vi "Lab Panel V5.22.vi"() -> ()   [LabVIEW 2013] (continued)
                      frame #0 {
                        n2184 = case shown="True" w3895 {
                          tunnel: w3894 -> [_ w3900]
                          tunnel: w3893 -> [_ w3899]
                          tunnel: w3892 -> [_ w3898]
                          tunnel: w3891 -> [_ w3896]
                          frame False {
                          }
                          frame True {
                            n2185 = Bundle(cluster=w3896, "amps"=w3900, "volts"=w3899, "pf"=w3898) -> (w3897:cluster{"amps":dbl, "volts":dbl, "pf":dbl})
                            n2186 = local write "ON L01-1"(w3897) -> ()
                          }
                        }
                      }
                      frame #1 {
                        n2187 = Unbundle(w3905) -> ("amps"=w3904:dbl, "volts"=w3903:dbl, "pf"=w3902:dbl)
                        n2188 = case shown="True" w3906 {
                          tunnel: w3913 -> [_ w3914]
                          tunnel: w3912 -> [_ w3952]
                          tunnel: w3911 -> [_ _]
                          tunnel: w3910 -> [_ _]
                          tunnel: w3909 -> [_ w3951]
                          tunnel: w3908 -> [_ w3950]
                          tunnel: w3907 -> [_ w3918]
                          tunnel: w3904 -> [_ w3915]
                          tunnel: w3903 -> [_ w3947]
                          tunnel: w3902 -> [_ w3946]
                          tunnel: w3901 -> [_ w3916]
                          frame False {
                          }
                          frame True {
                            n2189 = local read "TDMS LAB01-1"() -> (w3949:refnum<k34>)
                            n2190 = Build Array(w3947) -> (w3943:dbl[])
                            n2191 = Build Array(w3946) -> (w3942:dbl[])
                            n2192 = Build Array(w3951) -> (w3941:dbl[])
                            n2193 = Build Array(w3952) -> (w3940:dbl[])
                            n2194 = Build Array(w3915) -> (w3945:dbl[])
                            n2195 = Build Array(w3914) -> (w3944:dbl[])
                            n2196 = Build Array(w3950) -> (w3939:dbl[])
                            n2197 = Build Array("AMPS ON", "AMPS OFF", "VOLTS", "PF", "TEMP Live", "TEMP Neut", "CYCLE") -> (w3923:string[])
                            n2198 = Bundle By Name("Y"=w3945, "t0"=w3916) -> (w3938:waveform(dbl))  [unwired: 1 in]
                            n2199 = Bundle By Name("Y"=w3944, "t0"=w3916) -> (w3937:waveform(dbl))  [unwired: 1 in]
                            n2200 = Bundle By Name("Y"=w3943, "t0"=w3916) -> (w3936:waveform(dbl))  [unwired: 1 in]
                            n2201 = Bundle By Name("Y"=w3942, "t0"=w3916) -> (w3935:waveform(dbl))  [unwired: 1 in]
                            n2202 = Bundle By Name("Y"=w3941, "t0"=w3916) -> (w3934:waveform(dbl))  [unwired: 1 in]
                            n2203 = Bundle By Name("Y"=w3940, "t0"=w3916) -> (w3933:waveform(dbl))  [unwired: 1 in]
                            n2204 = Bundle By Name("Y"=w3939, "t0"=w3916) -> (w3932:waveform(dbl))  [unwired: 1 in]
                            n2205 = Build Array(w3938, w3937, w3936, w3935, w3934, w3933, w3932) -> (w3931:waveform(dbl)[])
                            n2206 = TDMS Write(0:w3949, 5:"TEST VALUES", 7:w3923, 9:w3931) -> (4:w3922:refnum<k34>, 6:w3921:string, 15:w3920:errorcluster)  [unwired: 2 in, 1 out]
                            n2207 = TDMS Write(0:w3922, 5:w3921, 7:"TIME", 9:w3918, 11:w3920) -> (15:w3917:errorcluster)  [unwired: 1 in, 3 out]
                            n2208 = local write "data file error"(w3917) -> ()
                          }
                        }
                      }
                    }
                  }
                }
              }
              frame #1 {
                n2209 = case shown="True" w3953 {
                  tunnel: w3957 -> [_ w3962]
                  tunnel: w3956 -> [_ w3961]
                  tunnel: w3955 -> [_ w3959]
                  tunnel: w3954 -> [_ w3958]
                  frame False {
                  }
                  frame True {
                    n2210 = local read "DISP LAB01-2"() -> (w3963:T4)
                    n2211 = local read "SIG LAB01-2"() -> (w3964:T2)
                    n2212 = local read "ON L01-2"() -> (w3960:cluster{"amps":dbl, "volts":dbl, "pf":dbl})
                    n2213 = Unbundle(w3964) -> ("AMPS"=w3970:dbl, "VOLTS"=w3968:dbl, "PF"=w3967:dbl, "Tmp Live"=w3966:dbl, "Tmp Neut"=w3969:dbl)
                    n2214 = Unbundle(w3963) -> ("CYCLE"=w3965:dbl)  [unwired: 2 out]
                    n2215 = stacked-sequence {
                      tunnel: w3970 -> [w3974 w3993]
                      tunnel: w3969 -> [_ w3992]
                      tunnel: w3968 -> [w3973 w3991]
                      tunnel: w3967 -> [w3972 w3990]
                      tunnel: w3966 -> [_ w3989]
                      tunnel: w3965 -> [_ w3988]
                      tunnel: w3962 -> [_ w3987]
                      tunnel: w3961 -> [w3975 _]
                      tunnel: w3960 -> [w3971 w3985]
                      tunnel: w3959 -> [_ w3986]
                      tunnel: w3958 -> [_ w3981]
                      frame #0 {
                        n2216 = case shown="True" w3975 {
                          tunnel: w3974 -> [_ w3980]
                          tunnel: w3973 -> [_ w3979]
                          tunnel: w3972 -> [_ w3978]
                          tunnel: w3971 -> [_ w3976]
                          frame False {
                          }
                          frame True {
                            n2217 = Bundle(cluster=w3976, "amps"=w3980, "volts"=w3979, "pf"=w3978) -> (w3977:cluster{"amps":dbl, "volts":dbl, "pf":dbl})
                            n2218 = local write "ON L01-2"(w3977) -> ()
                          }
                        }
                      }
                      frame #1 {
                        n2219 = Unbundle(w3985) -> ("amps"=w3984:dbl, "volts"=w3983:dbl, "pf"=w3982:dbl)
                        n2220 = case shown="True" w3986 {
                          tunnel: w3993 -> [_ w4025]
                          tunnel: w3992 -> [_ w4032]
                          tunnel: w3991 -> [_ _]
                          tunnel: w3990 -> [_ _]
                          tunnel: w3989 -> [_ w4031]
                          tunnel: w3988 -> [_ w4030]
                          tunnel: w3987 -> [_ w3995]
                          tunnel: w3984 -> [_ w4027]
                          tunnel: w3983 -> [_ w4026]
                          tunnel: w3982 -> [_ w4024]
                          tunnel: w3981 -> [_ w4016]
                          frame False {
                          }
                          frame True {
                            n2221 = local read "TDMS LAB01-2"() -> (w4029:refnum<k34>)
                            n2222 = Build Array(w4026) -> (w4021:dbl[])
                            n2223 = Build Array(w4024) -> (w4020:dbl[])
                            n2224 = Build Array(w4031) -> (w4019:dbl[])
                            n2225 = Build Array(w4032) -> (w4018:dbl[])
                            n2226 = Build Array(w4027) -> (w4023:dbl[])
                            n2227 = Build Array(w4025) -> (w4022:dbl[])
                            n2228 = Build Array(w4030) -> (w4017:dbl[])
                            n2229 = Build Array("AMPS ON", "AMPS OFF", "VOLTS", "PF", "TEMP Live", "TEMP Neut", "CYCLE") -> (w4000:string[])
                            n2230 = Bundle By Name("Y"=w4023, "t0"=w4016) -> (w4015:waveform(dbl))  [unwired: 1 in]
                            n2231 = Bundle By Name("Y"=w4022, "t0"=w4016) -> (w4014:waveform(dbl))  [unwired: 1 in]
                            n2232 = Bundle By Name("Y"=w4021, "t0"=w4016) -> (w4013:waveform(dbl))  [unwired: 1 in]
                            n2233 = Bundle By Name("Y"=w4020, "t0"=w4016) -> (w4012:waveform(dbl))  [unwired: 1 in]
                            n2234 = Bundle By Name("Y"=w4019, "t0"=w4016) -> (w4011:waveform(dbl))  [unwired: 1 in]
                            n2235 = Bundle By Name("Y"=w4018, "t0"=w4016) -> (w4010:waveform(dbl))  [unwired: 1 in]
                            n2236 = Bundle By Name("Y"=w4017, "t0"=w4016) -> (w4009:waveform(dbl))  [unwired: 1 in]
                            n2237 = Build Array(w4015, w4014, w4013, w4012, w4011, w4010, w4009) -> (w4008:waveform(dbl)[])
                            n2238 = TDMS Write(0:w4029, 5:"TEST VALUES", 7:w4000, 9:w4008) -> (4:w3999:refnum<k34>, 6:w3998:string, 15:w3997:errorcluster)  [unwired: 2 in, 1 out]
                            n2239 = TDMS Write(0:w3999, 5:w3998, 7:"TIME", 9:w3995, 11:w3997) -> (15:w3994:errorcluster)  [unwired: 1 in, 3 out]
                            n2240 = local write "data file error"(w3994) -> ()
                          }
                        }
                      }
                    }
                  }
                }
              }
              frame #2 {
                n2241 = case shown="True" w4033 {
                  tunnel: w4037 -> [_ w4042]
                  tunnel: w4036 -> [_ w4041]
                  tunnel: w4035 -> [_ w4039]
                  tunnel: w4034 -> [_ w4038]
                  frame False {
                  }
                  frame True {
                    n2242 = local read "DISP LAB02-1"() -> (w4043:T4)
                    n2243 = local read "SIG LAB02-1"() -> (w4044:T2)
                    n2244 = local read "ON L02-1"() -> (w4040:cluster{"amps":dbl, "volts":dbl, "pf":dbl})
                    n2245 = Unbundle(w4044) -> ("AMPS"=w4050:dbl, "VOLTS"=w4048:dbl, "PF"=w4047:dbl, "Tmp Live"=w4046:dbl, "Tmp Neut"=w4049:dbl)
                    n2246 = Unbundle(w4043) -> ("CYCLE"=w4045:dbl)  [unwired: 2 out]
                    n2247 = stacked-sequence {
                      tunnel: w4050 -> [w4054 w4073]
                      tunnel: w4049 -> [_ w4072]
                      tunnel: w4048 -> [w4053 w4071]
                      tunnel: w4047 -> [w4052 w4070]
                      tunnel: w4046 -> [_ w4069]
                      tunnel: w4045 -> [_ w4068]
                      tunnel: w4042 -> [_ w4067]
                      tunnel: w4041 -> [w4055 _]
                      tunnel: w4040 -> [w4051 w4065]
                      tunnel: w4039 -> [_ w4066]
                      tunnel: w4038 -> [_ w4061]
                      frame #0 {
                        n2248 = case shown="True" w4055 {
                          tunnel: w4054 -> [_ w4060]
                          tunnel: w4053 -> [_ w4059]
                          tunnel: w4052 -> [_ w4058]
                          tunnel: w4051 -> [_ w4056]
                          frame False {
                          }
                          frame True {
                            n2249 = Bundle(cluster=w4056, "amps"=w4060, "volts"=w4059, "pf"=w4058) -> (w4057:cluster{"amps":dbl, "volts":dbl, "pf":dbl})
                            n2250 = local write "ON L02-1"(w4057) -> ()
                          }
                        }
                      }
                      frame #1 {
                        n2251 = Unbundle(w4065) -> ("amps"=w4064:dbl, "volts"=w4063:dbl, "pf"=w4062:dbl)
                        n2252 = case shown="True" w4066 {
                          tunnel: w4073 -> [_ w4105]
                          tunnel: w4072 -> [_ w4112]
                          tunnel: w4071 -> [_ _]
                          tunnel: w4070 -> [_ _]
                          tunnel: w4069 -> [_ w4111]
                          tunnel: w4068 -> [_ w4110]
                          tunnel: w4067 -> [_ w4075]
                          tunnel: w4064 -> [_ w4107]
                          tunnel: w4063 -> [_ w4106]
                          tunnel: w4062 -> [_ w4104]
                          tunnel: w4061 -> [_ w4096]
                          frame False {
                          }
                          frame True {
                            n2253 = local read "TDMS LAB02-1"() -> (w4109:refnum<k34>)
                            n2254 = Build Array(w4106) -> (w4101:dbl[])
                            n2255 = Build Array(w4104) -> (w4100:dbl[])
                            n2256 = Build Array(w4111) -> (w4099:dbl[])
                            n2257 = Build Array(w4112) -> (w4098:dbl[])
                            n2258 = Build Array(w4107) -> (w4103:dbl[])
                            n2259 = Build Array(w4105) -> (w4102:dbl[])
                            n2260 = Build Array(w4110) -> (w4097:dbl[])
                            n2261 = Build Array("AMPS ON", "AMPS OFF", "VOLTS", "PF", "TEMP Live", "TEMP Neut", "CYCLE") -> (w4080:string[])
                            n2262 = Bundle By Name("Y"=w4103, "t0"=w4096) -> (w4095:waveform(dbl))  [unwired: 1 in]
                            n2263 = Bundle By Name("Y"=w4102, "t0"=w4096) -> (w4094:waveform(dbl))  [unwired: 1 in]
                            n2264 = Bundle By Name("Y"=w4101, "t0"=w4096) -> (w4093:waveform(dbl))  [unwired: 1 in]
                            n2265 = Bundle By Name("Y"=w4100, "t0"=w4096) -> (w4092:waveform(dbl))  [unwired: 1 in]
                            n2266 = Bundle By Name("Y"=w4099, "t0"=w4096) -> (w4091:waveform(dbl))  [unwired: 1 in]
                            n2267 = Bundle By Name("Y"=w4098, "t0"=w4096) -> (w4090:waveform(dbl))  [unwired: 1 in]
                            n2268 = Bundle By Name("Y"=w4097, "t0"=w4096) -> (w4089:waveform(dbl))  [unwired: 1 in]
                            n2269 = Build Array(w4095, w4094, w4093, w4092, w4091, w4090, w4089) -> (w4088:waveform(dbl)[])
                            n2270 = TDMS Write(0:w4109, 5:"TEST VALUES", 7:w4080, 9:w4088) -> (4:w4079:refnum<k34>, 6:w4078:string, 15:w4077:errorcluster)  [unwired: 2 in, 1 out]
                            n2271 = TDMS Write(0:w4079, 5:w4078, 7:"TIME", 9:w4075, 11:w4077) -> (15:w4074:errorcluster)  [unwired: 1 in, 3 out]
                            n2272 = local write "data file error"(w4074) -> ()
                          }
                        }
                      }
                    }
                  }
                }
              }
              frame #3 {
                n2273 = case shown="True" w4113 {
                  tunnel: w4117 -> [_ w4122]
                  tunnel: w4116 -> [_ w4121]
                  tunnel: w4115 -> [_ w4119]
                  tunnel: w4114 -> [_ w4118]
                  frame False {
                  }
                  frame True {
                    n2274 = local read "DISP LAB02-2"() -> (w4123:T4)
                    n2275 = local read "SIG LAB02-2"() -> (w4124:T2)
                    n2276 = local read "ON L02-2"() -> (w4120:cluster{"amps":dbl, "volts":dbl, "pf":dbl})
                    n2277 = Unbundle(w4124) -> ("AMPS"=w4130:dbl, "VOLTS"=w4128:dbl, "PF"=w4127:dbl, "Tmp Live"=w4126:dbl, "Tmp Neut"=w4129:dbl)
                    n2278 = Unbundle(w4123) -> ("CYCLE"=w4125:dbl)  [unwired: 2 out]
                    n2279 = stacked-sequence {
                      tunnel: w4130 -> [w4134 w4153]
                      tunnel: w4129 -> [_ w4152]
                      tunnel: w4128 -> [w4133 w4151]
                      tunnel: w4127 -> [w4132 w4150]
                      tunnel: w4126 -> [_ w4149]
                      tunnel: w4125 -> [_ w4148]
                      tunnel: w4122 -> [_ w4147]
                      tunnel: w4121 -> [w4135 _]
                      tunnel: w4120 -> [w4131 w4145]
                      tunnel: w4119 -> [_ w4146]
                      tunnel: w4118 -> [_ w4141]
                      frame #0 {
                        n2280 = case shown="True" w4135 {
                          tunnel: w4134 -> [_ w4140]
                          tunnel: w4133 -> [_ w4139]
                          tunnel: w4132 -> [_ w4138]
                          tunnel: w4131 -> [_ w4136]
                          frame False {
                          }
                          frame True {
                            n2281 = Bundle(cluster=w4136, "amps"=w4140, "volts"=w4139, "pf"=w4138) -> (w4137:cluster{"amps":dbl, "volts":dbl, "pf":dbl})
                            n2282 = local write "ON L02-2"(w4137) -> ()
                          }
                        }
                      }
                      frame #1 {
                        n2283 = Unbundle(w4145) -> ("amps"=w4144:dbl, "volts"=w4143:dbl, "pf"=w4142:dbl)
                        n2284 = case shown="True" w4146 {
                          tunnel: w4153 -> [_ w4185]
                          tunnel: w4152 -> [_ w4192]
                          tunnel: w4151 -> [_ _]
                          tunnel: w4150 -> [_ _]
                          tunnel: w4149 -> [_ w4191]
                          tunnel: w4148 -> [_ w4190]
                          tunnel: w4147 -> [_ w4155]
                          tunnel: w4144 -> [_ w4187]
                          tunnel: w4143 -> [_ w4186]
                          tunnel: w4142 -> [_ w4184]
                          tunnel: w4141 -> [_ w4176]
                          frame False {
                          }
                          frame True {
                            n2285 = local read "TDMS LAB02-2"() -> (w4189:refnum<k34>)
                            n2286 = Build Array(w4186) -> (w4181:dbl[])
                            n2287 = Build Array(w4184) -> (w4180:dbl[])
                            n2288 = Build Array(w4191) -> (w4179:dbl[])
                            n2289 = Build Array(w4192) -> (w4178:dbl[])
                            n2290 = Build Array(w4187) -> (w4183:dbl[])
                            n2291 = Build Array(w4185) -> (w4182:dbl[])
                            n2292 = Build Array(w4190) -> (w4177:dbl[])
                            n2293 = Build Array("AMPS ON", "AMPS OFF", "VOLTS", "PF", "TEMP Live", "TEMP Neut", "CYCLE") -> (w4160:string[])
                            n2294 = Bundle By Name("Y"=w4183, "t0"=w4176) -> (w4175:waveform(dbl))  [unwired: 1 in]
                            n2295 = Bundle By Name("Y"=w4182, "t0"=w4176) -> (w4174:waveform(dbl))  [unwired: 1 in]
                            n2296 = Bundle By Name("Y"=w4181, "t0"=w4176) -> (w4173:waveform(dbl))  [unwired: 1 in]
                            n2297 = Bundle By Name("Y"=w4180, "t0"=w4176) -> (w4172:waveform(dbl))  [unwired: 1 in]
                            n2298 = Bundle By Name("Y"=w4179, "t0"=w4176) -> (w4171:waveform(dbl))  [unwired: 1 in]
                            n2299 = Bundle By Name("Y"=w4178, "t0"=w4176) -> (w4170:waveform(dbl))  [unwired: 1 in]
                            n2300 = Bundle By Name("Y"=w4177, "t0"=w4176) -> (w4169:waveform(dbl))  [unwired: 1 in]
                            n2301 = Build Array(w4175, w4174, w4173, w4172, w4171, w4170, w4169) -> (w4168:waveform(dbl)[])
                            n2302 = TDMS Write(0:w4189, 5:"TEST VALUES", 7:w4160, 9:w4168) -> (4:w4159:refnum<k34>, 6:w4158:string, 15:w4157:errorcluster)  [unwired: 2 in, 1 out]
                            n2303 = TDMS Write(0:w4159, 5:w4158, 7:"TIME", 9:w4155, 11:w4157) -> (15:w4154:errorcluster)  [unwired: 1 in, 3 out]
                            n2304 = local write "data file error"(w4154) -> ()
                          }
                        }
                      }
                    }
                  }
                }
              }
              frame #4 {
                n2305 = case shown="True" w4193 {
                  tunnel: w4197 -> [_ w4202]
                  tunnel: w4196 -> [_ w4201]
                  tunnel: w4195 -> [_ w4199]
                  tunnel: w4194 -> [_ w4198]
                  frame False {
                  }
                  frame True {
                    n2306 = local read "DISP LAB03-1"() -> (w4203:T4)
                    n2307 = local read "SIG LAB03-1"() -> (w4204:T2)
                    n2308 = local read "ON L03-1"() -> (w4200:cluster{"amps":dbl, "volts":dbl, "pf":dbl})
                    n2309 = Unbundle(w4204) -> ("AMPS"=w4210:dbl, "VOLTS"=w4208:dbl, "PF"=w4207:dbl, "Tmp Live"=w4206:dbl, "Tmp Neut"=w4209:dbl)
                    n2310 = Unbundle(w4203) -> ("CYCLE"=w4205:dbl)  [unwired: 2 out]
                    n2311 = stacked-sequence {
                      tunnel: w4210 -> [w4214 w4233]
                      tunnel: w4209 -> [_ w4232]
                      tunnel: w4208 -> [w4213 w4231]
                      tunnel: w4207 -> [w4212 w4230]
                      tunnel: w4206 -> [_ w4229]
                      tunnel: w4205 -> [_ w4228]
                      tunnel: w4202 -> [_ w4227]
                      tunnel: w4201 -> [w4215 _]
                      tunnel: w4200 -> [w4211 w4225]
                      tunnel: w4199 -> [_ w4226]
                      tunnel: w4198 -> [_ w4221]
                      frame #0 {
                        n2312 = case shown="True" w4215 {
                          tunnel: w4214 -> [_ w4220]
                          tunnel: w4213 -> [_ w4219]
                          tunnel: w4212 -> [_ w4218]
                          tunnel: w4211 -> [_ w4216]
                          frame False {
                          }
                          frame True {
                            n2313 = Bundle(cluster=w4216, "amps"=w4220, "volts"=w4219, "pf"=w4218) -> (w4217:cluster{"amps":dbl, "volts":dbl, "pf":dbl})
                            n2314 = local write "ON L03-1"(w4217) -> ()
                          }
                        }
                      }
                      frame #1 {
                        n2315 = Unbundle(w4225) -> ("amps"=w4224:dbl, "volts"=w4223:dbl, "pf"=w4222:dbl)
                        n2316 = case shown="True" w4226 {
                          tunnel: w4233 -> [_ w4265]
                          tunnel: w4232 -> [_ w4272]
                          tunnel: w4231 -> [_ _]
                          tunnel: w4230 -> [_ _]
                          tunnel: w4229 -> [_ w4271]
                          tunnel: w4228 -> [_ w4270]
                          tunnel: w4227 -> [_ w4235]
                          tunnel: w4224 -> [_ w4267]
                          tunnel: w4223 -> [_ w4266]
                          tunnel: w4222 -> [_ w4264]
                          tunnel: w4221 -> [_ w4256]
                          frame False {
                          }
                          frame True {
                            n2317 = local read "TDMS LAB03-1"() -> (w4269:refnum<k34>)
                            n2318 = Build Array(w4266) -> (w4261:dbl[])
                            n2319 = Build Array(w4264) -> (w4260:dbl[])
                            n2320 = Build Array(w4271) -> (w4259:dbl[])
                            n2321 = Build Array(w4272) -> (w4258:dbl[])
                            n2322 = Build Array(w4267) -> (w4263:dbl[])
                            n2323 = Build Array(w4265) -> (w4262:dbl[])
                            n2324 = Build Array(w4270) -> (w4257:dbl[])
                            n2325 = Build Array("AMPS ON", "AMPS OFF", "VOLTS", "PF", "TEMP Live", "TEMP Neut", "CYCLE") -> (w4240:string[])
                            n2326 = Bundle By Name("Y"=w4263, "t0"=w4256) -> (w4255:waveform(dbl))  [unwired: 1 in]
                            n2327 = Bundle By Name("Y"=w4262, "t0"=w4256) -> (w4254:waveform(dbl))  [unwired: 1 in]
                            n2328 = Bundle By Name("Y"=w4261, "t0"=w4256) -> (w4253:waveform(dbl))  [unwired: 1 in]
                            n2329 = Bundle By Name("Y"=w4260, "t0"=w4256) -> (w4252:waveform(dbl))  [unwired: 1 in]
                            n2330 = Bundle By Name("Y"=w4259, "t0"=w4256) -> (w4251:waveform(dbl))  [unwired: 1 in]
                            n2331 = Bundle By Name("Y"=w4258, "t0"=w4256) -> (w4250:waveform(dbl))  [unwired: 1 in]
                            n2332 = Bundle By Name("Y"=w4257, "t0"=w4256) -> (w4249:waveform(dbl))  [unwired: 1 in]
                            n2333 = Build Array(w4255, w4254, w4253, w4252, w4251, w4250, w4249) -> (w4248:waveform(dbl)[])
                            n2334 = TDMS Write(0:w4269, 5:"TEST VALUES", 7:w4240, 9:w4248) -> (4:w4239:refnum<k34>, 6:w4238:string, 15:w4237:errorcluster)  [unwired: 2 in, 1 out]
                            n2335 = TDMS Write(0:w4239, 5:w4238, 7:"TIME", 9:w4235, 11:w4237) -> (15:w4234:errorcluster)  [unwired: 1 in, 3 out]
                            n2336 = local write "data file error"(w4234) -> ()
                          }
                        }
                      }
                    }
                  }
                }
              }
              frame #5 {
                n2337 = case shown="True" w4273 {
                  tunnel: w4277 -> [_ w4282]
                  tunnel: w4276 -> [_ w4281]
                  tunnel: w4275 -> [_ w4279]
                  tunnel: w4274 -> [_ w4278]
                  frame False {
                  }
                  frame True {
                    n2338 = local read "DISP LAB03-2"() -> (w4283:T4)
                    n2339 = local read "SIG LAB03-2"() -> (w4284:T2)
                    n2340 = local read "ON L03-2"() -> (w4280:cluster{"amps":dbl, "volts":dbl, "pf":dbl})
                    n2341 = Unbundle(w4284) -> ("AMPS"=w4290:dbl, "VOLTS"=w4288:dbl, "PF"=w4287:dbl, "Tmp Live"=w4286:dbl, "Tmp Neut"=w4289:dbl)
                    n2342 = Unbundle(w4283) -> ("CYCLE"=w4285:dbl)  [unwired: 2 out]
                    n2343 = stacked-sequence {
                      tunnel: w4290 -> [w4294 w4313]
                      tunnel: w4289 -> [_ w4312]
                      tunnel: w4288 -> [w4293 w4311]
                      tunnel: w4287 -> [w4292 w4310]
                      tunnel: w4286 -> [_ w4309]
                      tunnel: w4285 -> [_ w4308]
                      tunnel: w4282 -> [_ w4307]
                      tunnel: w4281 -> [w4295 _]
                      tunnel: w4280 -> [w4291 w4305]
                      tunnel: w4279 -> [_ w4306]
                      tunnel: w4278 -> [_ w4301]
                      frame #0 {
                        n2344 = case shown="True" w4295 {
                          tunnel: w4294 -> [_ w4300]
                          tunnel: w4293 -> [_ w4299]
                          tunnel: w4292 -> [_ w4298]
                          tunnel: w4291 -> [_ w4296]
                          frame False {
                          }
                          frame True {
                            n2345 = Bundle(cluster=w4296, "amps"=w4300, "volts"=w4299, "pf"=w4298) -> (w4297:cluster{"amps":dbl, "volts":dbl, "pf":dbl})
                            n2346 = local write "ON L03-2"(w4297) -> ()
                          }
                        }
                      }
                      frame #1 {
                        n2347 = Unbundle(w4305) -> ("amps"=w4304:dbl, "volts"=w4303:dbl, "pf"=w4302:dbl)
                        n2348 = case shown="True" w4306 {
                          tunnel: w4313 -> [_ w4345]
                          tunnel: w4312 -> [_ w4352]
                          tunnel: w4311 -> [_ _]
                          tunnel: w4310 -> [_ _]
                          tunnel: w4309 -> [_ w4351]
                          tunnel: w4308 -> [_ w4350]
                          tunnel: w4307 -> [_ w4315]
                          tunnel: w4304 -> [_ w4347]
                          tunnel: w4303 -> [_ w4346]
                          tunnel: w4302 -> [_ w4344]
                          tunnel: w4301 -> [_ w4336]
                          frame False {
                          }
                          frame True {
                            n2349 = local read "TDMS LAB03-2"() -> (w4349:refnum<k34>)
                            n2350 = Build Array(w4346) -> (w4341:dbl[])
                            n2351 = Build Array(w4344) -> (w4340:dbl[])
                            n2352 = Build Array(w4351) -> (w4339:dbl[])
                            n2353 = Build Array(w4352) -> (w4338:dbl[])
                            n2354 = Build Array(w4347) -> (w4343:dbl[])
                            n2355 = Build Array(w4345) -> (w4342:dbl[])
                            n2356 = Build Array(w4350) -> (w4337:dbl[])
                            n2357 = Build Array("AMPS ON", "AMPS OFF", "VOLTS", "PF", "TEMP Live", "TEMP Neut", "CYCLE") -> (w4320:string[])
                            n2358 = Bundle By Name("Y"=w4343, "t0"=w4336) -> (w4335:waveform(dbl))  [unwired: 1 in]
                            n2359 = Bundle By Name("Y"=w4342, "t0"=w4336) -> (w4334:waveform(dbl))  [unwired: 1 in]
                            n2360 = Bundle By Name("Y"=w4341, "t0"=w4336) -> (w4333:waveform(dbl))  [unwired: 1 in]
                            n2361 = Bundle By Name("Y"=w4340, "t0"=w4336) -> (w4332:waveform(dbl))  [unwired: 1 in]
                            n2362 = Bundle By Name("Y"=w4339, "t0"=w4336) -> (w4331:waveform(dbl))  [unwired: 1 in]
                            n2363 = Bundle By Name("Y"=w4338, "t0"=w4336) -> (w4330:waveform(dbl))  [unwired: 1 in]
                            n2364 = Bundle By Name("Y"=w4337, "t0"=w4336) -> (w4329:waveform(dbl))  [unwired: 1 in]
                            n2365 = Build Array(w4335, w4334, w4333, w4332, w4331, w4330, w4329) -> (w4328:waveform(dbl)[])
                            n2366 = TDMS Write(0:w4349, 5:"TEST VALUES", 7:w4320, 9:w4328) -> (4:w4319:refnum<k34>, 6:w4318:string, 15:w4317:errorcluster)  [unwired: 2 in, 1 out]
                            n2367 = TDMS Write(0:w4319, 5:w4318, 7:"TIME", 9:w4315, 11:w4317) -> (15:w4314:errorcluster)  [unwired: 1 in, 3 out]
                            n2368 = local write "data file error"(w4314) -> ()
                          }
                        }
                      }
                    }
                  }
                }
              }
              frame #6 {
                n2369 = case shown="True" w4353 {
                  tunnel: w4357 -> [_ w4362]
                  tunnel: w4356 -> [_ w4361]
                  tunnel: w4355 -> [_ w4359]
                  tunnel: w4354 -> [_ w4358]
                  frame False {
                  }
                  frame True {
                    n2370 = local read "DISP LAB04-1"() -> (w4363:T4)
                    n2371 = local read "SIG LAB04-1"() -> (w4364:T2)
                    n2372 = local read "ON L04-1"() -> (w4360:cluster{"amps":dbl, "volts":dbl, "pf":dbl})
                    n2373 = Unbundle(w4364) -> ("AMPS"=w4370:dbl, "VOLTS"=w4368:dbl, "PF"=w4367:dbl, "Tmp Live"=w4366:dbl, "Tmp Neut"=w4369:dbl)
                    n2374 = Unbundle(w4363) -> ("CYCLE"=w4365:dbl)  [unwired: 2 out]
                    n2375 = stacked-sequence {
                      tunnel: w4370 -> [w4374 w4393]
                      tunnel: w4369 -> [_ w4392]
                      tunnel: w4368 -> [w4373 w4391]
                      tunnel: w4367 -> [w4372 w4390]
                      tunnel: w4366 -> [_ w4389]
                      tunnel: w4365 -> [_ w4388]
                      tunnel: w4362 -> [_ w4387]
                      tunnel: w4361 -> [w4375 _]
                      tunnel: w4360 -> [w4371 w4385]
                      tunnel: w4359 -> [_ w4386]
                      tunnel: w4358 -> [_ w4381]
                      frame #0 {
                        n2376 = case shown="True" w4375 {
                          tunnel: w4374 -> [_ w4380]
                          tunnel: w4373 -> [_ w4379]
                          tunnel: w4372 -> [_ w4378]
                          tunnel: w4371 -> [_ w4376]
                          frame False {
                          }
                          frame True {
                            n2377 = Bundle(cluster=w4376, "amps"=w4380, "volts"=w4379, "pf"=w4378) -> (w4377:cluster{"amps":dbl, "volts":dbl, "pf":dbl})
                            n2378 = local write "ON L04-1"(w4377) -> ()
                          }
                        }
                      }
                      frame #1 {
                        n2379 = Unbundle(w4385) -> ("amps"=w4384:dbl, "volts"=w4383:dbl, "pf"=w4382:dbl)
                        n2380 = case shown="True" w4386 {
                          tunnel: w4393 -> [_ w4425]
                          tunnel: w4392 -> [_ w4432]
                          tunnel: w4391 -> [_ _]
                          tunnel: w4390 -> [_ _]
                          tunnel: w4389 -> [_ w4431]
                          tunnel: w4388 -> [_ w4430]
                          tunnel: w4387 -> [_ w4395]
                          tunnel: w4384 -> [_ w4427]
                          tunnel: w4383 -> [_ w4426]
                          tunnel: w4382 -> [_ w4424]
                          tunnel: w4381 -> [_ w4416]
                          frame False {
                          }
                          frame True {
                            n2381 = local read "TDMS LAB04-1"() -> (w4429:refnum<k34>)
                            n2382 = Build Array(w4426) -> (w4421:dbl[])
                            n2383 = Build Array(w4424) -> (w4420:dbl[])
                            n2384 = Build Array(w4431) -> (w4419:dbl[])
                            n2385 = Build Array(w4432) -> (w4418:dbl[])
                            n2386 = Build Array(w4427) -> (w4423:dbl[])
                            n2387 = Build Array(w4425) -> (w4422:dbl[])
                            n2388 = Build Array(w4430) -> (w4417:dbl[])
                            n2389 = Build Array("AMPS ON", "AMPS OFF", "VOLTS", "PF", "TEMP Live", "TEMP Neut", "CYCLE") -> (w4400:string[])
                            n2390 = Bundle By Name("Y"=w4423, "t0"=w4416) -> (w4415:waveform(dbl))  [unwired: 1 in]
                            n2391 = Bundle By Name("Y"=w4422, "t0"=w4416) -> (w4414:waveform(dbl))  [unwired: 1 in]
                            n2392 = Bundle By Name("Y"=w4421, "t0"=w4416) -> (w4413:waveform(dbl))  [unwired: 1 in]
                            n2393 = Bundle By Name("Y"=w4420, "t0"=w4416) -> (w4412:waveform(dbl))  [unwired: 1 in]
                            n2394 = Bundle By Name("Y"=w4419, "t0"=w4416) -> (w4411:waveform(dbl))  [unwired: 1 in]
                            n2395 = Bundle By Name("Y"=w4418, "t0"=w4416) -> (w4410:waveform(dbl))  [unwired: 1 in]
                            n2396 = Bundle By Name("Y"=w4417, "t0"=w4416) -> (w4409:waveform(dbl))  [unwired: 1 in]
                            n2397 = Build Array(w4415, w4414, w4413, w4412, w4411, w4410, w4409) -> (w4408:waveform(dbl)[])
                            n2398 = TDMS Write(0:w4429, 5:"TEST VALUES", 7:w4400, 9:w4408) -> (4:w4399:refnum<k34>, 6:w4398:string, 15:w4397:errorcluster)  [unwired: 2 in, 1 out]
                            n2399 = TDMS Write(0:w4399, 5:w4398, 7:"TIME", 9:w4395, 11:w4397) -> (15:w4394:errorcluster)  [unwired: 1 in, 3 out]
                            n2400 = local write "data file error"(w4394) -> ()
                          }
                        }
                      }
                    }
                  }
                }
              }
              frame #7 {
                n2401 = case shown="True" w4433 {
                  tunnel: w4437 -> [_ w4442]
                  tunnel: w4436 -> [_ w4441]
                  tunnel: w4435 -> [_ w4439]
                  tunnel: w4434 -> [_ w4438]
                  frame False {
                  }
                  frame True {
                    n2402 = local read "DISP LAB04-2"() -> (w4443:T4)
                    n2403 = local read "SIG LAB04-2"() -> (w4444:T2)
                    n2404 = local read "ON L04-2"() -> (w4440:cluster{"amps":dbl, "volts":dbl, "pf":dbl})
                    n2405 = Unbundle(w4444) -> ("AMPS"=w4450:dbl, "VOLTS"=w4448:dbl, "PF"=w4447:dbl, "Tmp Live"=w4446:dbl, "Tmp Neut"=w4449:dbl)
                    n2406 = Unbundle(w4443) -> ("CYCLE"=w4445:dbl)  [unwired: 2 out]
                    n2407 = stacked-sequence {
                      tunnel: w4450 -> [w4454 w4473]
                      tunnel: w4449 -> [_ w4472]
                      tunnel: w4448 -> [w4453 w4471]
                      tunnel: w4447 -> [w4452 w4470]
                      tunnel: w4446 -> [_ w4469]
                      tunnel: w4445 -> [_ w4468]
                      tunnel: w4442 -> [_ w4467]
                      tunnel: w4441 -> [w4455 _]
                      tunnel: w4440 -> [w4451 w4465]
                      tunnel: w4439 -> [_ w4466]
                      tunnel: w4438 -> [_ w4461]
                      frame #0 {
                        n2408 = case shown="True" w4455 {
                          tunnel: w4454 -> [_ w4460]
                          tunnel: w4453 -> [_ w4459]
                          tunnel: w4452 -> [_ w4458]
                          tunnel: w4451 -> [_ w4456]
                          frame False {
                          }
                          frame True {
                            n2409 = Bundle(cluster=w4456, "amps"=w4460, "volts"=w4459, "pf"=w4458) -> (w4457:cluster{"amps":dbl, "volts":dbl, "pf":dbl})
                            n2410 = local write "ON L04-2"(w4457) -> ()
                          }
                        }
                      }
                      frame #1 {
                        n2411 = Unbundle(w4465) -> ("amps"=w4464:dbl, "volts"=w4463:dbl, "pf"=w4462:dbl)
                        n2412 = case shown="True" w4466 {
                          tunnel: w4473 -> [_ w4505]
                          tunnel: w4472 -> [_ w4512]
                          tunnel: w4471 -> [_ _]
                          tunnel: w4470 -> [_ _]
                          tunnel: w4469 -> [_ w4511]
                          tunnel: w4468 -> [_ w4510]
                          tunnel: w4467 -> [_ w4475]
                          tunnel: w4464 -> [_ w4507]
                          tunnel: w4463 -> [_ w4506]
                          tunnel: w4462 -> [_ w4504]
                          tunnel: w4461 -> [_ w4496]
                          frame False {
                          }
                          frame True {
                            n2413 = local read "TDMS LAB04-2"() -> (w4509:refnum<k34>)
                            n2414 = Build Array(w4506) -> (w4501:dbl[])
                            n2415 = Build Array(w4504) -> (w4500:dbl[])
                            n2416 = Build Array(w4511) -> (w4499:dbl[])
                            n2417 = Build Array(w4512) -> (w4498:dbl[])
                            n2418 = Build Array(w4507) -> (w4503:dbl[])
                            n2419 = Build Array(w4505) -> (w4502:dbl[])
                            n2420 = Build Array(w4510) -> (w4497:dbl[])
                            n2421 = Build Array("AMPS ON", "AMPS OFF", "VOLTS", "PF", "TEMP Live", "TEMP Neut", "CYCLE") -> (w4480:string[])
                            n2422 = Bundle By Name("Y"=w4503, "t0"=w4496) -> (w4495:waveform(dbl))  [unwired: 1 in]
                            n2423 = Bundle By Name("Y"=w4502, "t0"=w4496) -> (w4494:waveform(dbl))  [unwired: 1 in]
                            n2424 = Bundle By Name("Y"=w4501, "t0"=w4496) -> (w4493:waveform(dbl))  [unwired: 1 in]
                            n2425 = Bundle By Name("Y"=w4500, "t0"=w4496) -> (w4492:waveform(dbl))  [unwired: 1 in]
                            n2426 = Bundle By Name("Y"=w4499, "t0"=w4496) -> (w4491:waveform(dbl))  [unwired: 1 in]
                            n2427 = Bundle By Name("Y"=w4498, "t0"=w4496) -> (w4490:waveform(dbl))  [unwired: 1 in]
                            n2428 = Bundle By Name("Y"=w4497, "t0"=w4496) -> (w4489:waveform(dbl))  [unwired: 1 in]
                            n2429 = Build Array(w4495, w4494, w4493, w4492, w4491, w4490, w4489) -> (w4488:waveform(dbl)[])
                            n2430 = TDMS Write(0:w4509, 5:"TEST VALUES", 7:w4480, 9:w4488) -> (4:w4479:refnum<k34>, 6:w4478:string, 15:w4477:errorcluster)  [unwired: 2 in, 1 out]
                            n2431 = TDMS Write(0:w4479, 5:w4478, 7:"TIME", 9:w4475, 11:w4477) -> (15:w4474:errorcluster)  [unwired: 1 in, 3 out]
                            n2432 = local write "data file error"(w4474) -> ()
                          }
                        }
                      }
                    }
                  }
                }
              }
              frame #8 {
                n2433 = case shown="True" w4513 {
                  tunnel: w4517 -> [_ w4522]
                  tunnel: w4516 -> [_ w4521]
                  tunnel: w4515 -> [_ w4519]
                  tunnel: w4514 -> [_ w4518]
                  frame False {
                  }
                  frame True {
                    n2434 = local read "DISP LAB05-1"() -> (w4523:T4)
                    n2435 = local read "SIG LAB05-1"() -> (w4524:T2)
                    n2436 = local read "ON L05-1"() -> (w4520:cluster{"amps":dbl, "volts":dbl, "pf":dbl})
                    n2437 = Unbundle(w4524) -> ("AMPS"=w4530:dbl, "VOLTS"=w4528:dbl, "PF"=w4527:dbl, "Tmp Live"=w4526:dbl, "Tmp Neut"=w4529:dbl)
                    n2438 = Unbundle(w4523) -> ("CYCLE"=w4525:dbl)  [unwired: 2 out]
                    n2439 = stacked-sequence {
                      tunnel: w4530 -> [w4534 w4553]
                      tunnel: w4529 -> [_ w4552]
                      tunnel: w4528 -> [w4533 w4551]
                      tunnel: w4527 -> [w4532 w4550]
                      tunnel: w4526 -> [_ w4549]
                      tunnel: w4525 -> [_ w4548]
                      tunnel: w4522 -> [_ w4547]
                      tunnel: w4521 -> [w4535 _]
                      tunnel: w4520 -> [w4531 w4545]
                      tunnel: w4519 -> [_ w4546]
                      tunnel: w4518 -> [_ w4541]
                      frame #0 {
                        n2440 = case shown="True" w4535 {
                          tunnel: w4534 -> [_ w4540]
                          tunnel: w4533 -> [_ w4539]
                          tunnel: w4532 -> [_ w4538]
                          tunnel: w4531 -> [_ w4536]
                          frame False {
                          }
                          frame True {
                            n2441 = Bundle(cluster=w4536, "amps"=w4540, "volts"=w4539, "pf"=w4538) -> (w4537:cluster{"amps":dbl, "volts":dbl, "pf":dbl})
                            n2442 = local write "ON L05-1"(w4537) -> ()
                          }
                        }
                      }
                      frame #1 {
                        n2443 = Unbundle(w4545) -> ("amps"=w4544:dbl, "volts"=w4543:dbl, "pf"=w4542:dbl)
                        n2444 = case shown="True" w4546 {
                          tunnel: w4553 -> [_ w4585]
                          tunnel: w4552 -> [_ w4592]
                          tunnel: w4551 -> [_ _]
                          tunnel: w4550 -> [_ _]
                          tunnel: w4549 -> [_ w4591]
                          tunnel: w4548 -> [_ w4590]
                          tunnel: w4547 -> [_ w4555]
                          tunnel: w4544 -> [_ w4587]
                          tunnel: w4543 -> [_ w4586]
                          tunnel: w4542 -> [_ w4584]
                          tunnel: w4541 -> [_ w4576]
                          frame False {
                          }
                          frame True {
                            n2445 = local read "TDMS LAB05-1"() -> (w4589:refnum<k34>)
                            n2446 = Build Array(w4586) -> (w4581:dbl[])
                            n2447 = Build Array(w4584) -> (w4580:dbl[])
                            n2448 = Build Array(w4591) -> (w4579:dbl[])
                            n2449 = Build Array(w4592) -> (w4578:dbl[])
                            n2450 = Build Array(w4587) -> (w4583:dbl[])
                            n2451 = Build Array(w4585) -> (w4582:dbl[])
                            n2452 = Build Array(w4590) -> (w4577:dbl[])
                            n2453 = Build Array("AMPS ON", "AMPS OFF", "VOLTS", "PF", "TEMP Live", "TEMP Neut", "CYCLE") -> (w4560:string[])
                            n2454 = Bundle By Name("Y"=w4583, "t0"=w4576) -> (w4575:waveform(dbl))  [unwired: 1 in]
                            n2455 = Bundle By Name("Y"=w4582, "t0"=w4576) -> (w4574:waveform(dbl))  [unwired: 1 in]
                            n2456 = Bundle By Name("Y"=w4581, "t0"=w4576) -> (w4573:waveform(dbl))  [unwired: 1 in]
                            n2457 = Bundle By Name("Y"=w4580, "t0"=w4576) -> (w4572:waveform(dbl))  [unwired: 1 in]
                            n2458 = Bundle By Name("Y"=w4579, "t0"=w4576) -> (w4571:waveform(dbl))  [unwired: 1 in]
                            n2459 = Bundle By Name("Y"=w4578, "t0"=w4576) -> (w4570:waveform(dbl))  [unwired: 1 in]
                            n2460 = Bundle By Name("Y"=w4577, "t0"=w4576) -> (w4569:waveform(dbl))  [unwired: 1 in]
                            n2461 = Build Array(w4575, w4574, w4573, w4572, w4571, w4570, w4569) -> (w4568:waveform(dbl)[])
                            n2462 = TDMS Write(0:w4589, 5:"TEST VALUES", 7:w4560, 9:w4568) -> (4:w4559:refnum<k34>, 6:w4558:string, 15:w4557:errorcluster)  [unwired: 2 in, 1 out]
                            n2463 = TDMS Write(0:w4559, 5:w4558, 7:"TIME", 9:w4555, 11:w4557) -> (15:w4554:errorcluster)  [unwired: 1 in, 3 out]
                            n2464 = local write "data file error"(w4554) -> ()
                          }
                        }
                      }
                    }
                  }
                }
              }
              frame #9 {
                n2465 = case shown="True" w4593 {
                  tunnel: w4597 -> [_ w4602]
                  tunnel: w4596 -> [_ w4601]
                  tunnel: w4595 -> [_ w4599]
                  tunnel: w4594 -> [_ w4598]
                  frame False {
                  }
                  frame True {
                    n2466 = local read "DISP LAB05-2"() -> (w4603:T4)
                    n2467 = local read "SIG LAB05-2"() -> (w4604:T2)
                    n2468 = local read "ON L05-2"() -> (w4600:cluster{"amps":dbl, "volts":dbl, "pf":dbl})
                    n2469 = Unbundle(w4604) -> ("AMPS"=w4610:dbl, "VOLTS"=w4608:dbl, "PF"=w4607:dbl, "Tmp Live"=w4606:dbl, "Tmp Neut"=w4609:dbl)
                    n2470 = Unbundle(w4603) -> ("CYCLE"=w4605:dbl)  [unwired: 2 out]
                    n2471 = stacked-sequence {
                      tunnel: w4610 -> [w4614 w4633]
                      tunnel: w4609 -> [_ w4632]
                      tunnel: w4608 -> [w4613 w4631]
                      tunnel: w4607 -> [w4612 w4630]
                      tunnel: w4606 -> [_ w4629]
                      tunnel: w4605 -> [_ w4628]
                      tunnel: w4602 -> [_ w4627]
                      tunnel: w4601 -> [w4615 _]
                      tunnel: w4600 -> [w4611 w4625]
                      tunnel: w4599 -> [_ w4626]
                      tunnel: w4598 -> [_ w4621]
                      frame #0 {
                        n2472 = case shown="True" w4615 {
                          tunnel: w4614 -> [_ w4620]
                          tunnel: w4613 -> [_ w4619]
                          tunnel: w4612 -> [_ w4618]
                          tunnel: w4611 -> [_ w4616]
                          frame False {
                          }
                          frame True {
                            n2473 = Bundle(cluster=w4616, "amps"=w4620, "volts"=w4619, "pf"=w4618) -> (w4617:cluster{"amps":dbl, "volts":dbl, "pf":dbl})
                            n2474 = local write "ON L05-2"(w4617) -> ()
                          }
                        }
                      }
                      frame #1 {
                        n2475 = Unbundle(w4625) -> ("amps"=w4624:dbl, "volts"=w4623:dbl, "pf"=w4622:dbl)
                        n2476 = case shown="True" w4626 {
                          tunnel: w4633 -> [_ w4665]
                          tunnel: w4632 -> [_ w4672]
                          tunnel: w4631 -> [_ _]
                          tunnel: w4630 -> [_ _]
                          tunnel: w4629 -> [_ w4671]
                          tunnel: w4628 -> [_ w4670]
                          tunnel: w4627 -> [_ w4635]
                          tunnel: w4624 -> [_ w4667]
                          tunnel: w4623 -> [_ w4666]
                          tunnel: w4622 -> [_ w4664]
                          tunnel: w4621 -> [_ w4656]
                          frame False {
                          }
                          frame True {
                            n2477 = local read "TDMS LAB05-2"() -> (w4669:refnum<k34>)
                            n2478 = Build Array(w4666) -> (w4661:dbl[])
                            n2479 = Build Array(w4664) -> (w4660:dbl[])
                            n2480 = Build Array(w4671) -> (w4659:dbl[])
                            n2481 = Build Array(w4672) -> (w4658:dbl[])
                            n2482 = Build Array(w4667) -> (w4663:dbl[])
                            n2483 = Build Array(w4665) -> (w4662:dbl[])
                            n2484 = Build Array(w4670) -> (w4657:dbl[])
                            n2485 = Build Array("AMPS ON", "AMPS OFF", "VOLTS", "PF", "TEMP Live", "TEMP Neut", "CYCLE") -> (w4640:string[])
                            n2486 = Bundle By Name("Y"=w4663, "t0"=w4656) -> (w4655:waveform(dbl))  [unwired: 1 in]
                            n2487 = Bundle By Name("Y"=w4662, "t0"=w4656) -> (w4654:waveform(dbl))  [unwired: 1 in]
                            n2488 = Bundle By Name("Y"=w4661, "t0"=w4656) -> (w4653:waveform(dbl))  [unwired: 1 in]
                            n2489 = Bundle By Name("Y"=w4660, "t0"=w4656) -> (w4652:waveform(dbl))  [unwired: 1 in]
                            n2490 = Bundle By Name("Y"=w4659, "t0"=w4656) -> (w4651:waveform(dbl))  [unwired: 1 in]
